vi "DO State Machine.vi"(0 "DO in":bool, 5 "Set":bool, 7 "Time uSec":u32) -> (4 "DO out":bool)   [LabVIEW 2019]
uses:
  <vilib>/rvi/Emulation/niFpgaGetClockAttributes.vi
  <vilib>/rvi/Emulation/niFpgaSctlEmulationGetInTimedLoop.vi
  <vilib>/rvi/Emulation/niFpgaEmulationReportErrorSimple.vi
  <vilib>/rvi/Emulation/niFpgaCriticalErrorInLSC.vi
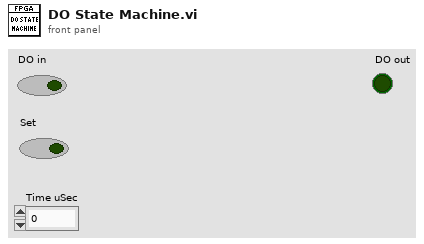
[diagram p1: front panel]
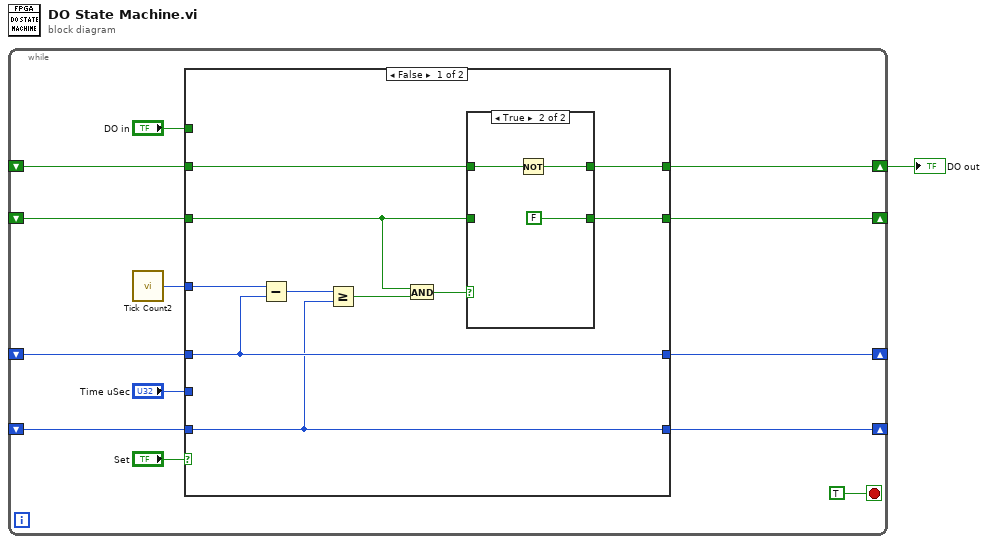
[diagram p0: block diagram]
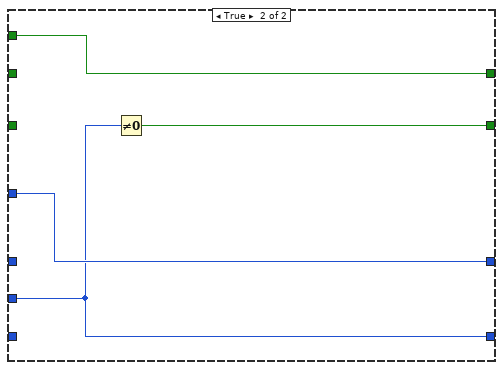
[diagram p3: hidden frame]
diagram:
  n1 = while {
    shift-right: [w9] -> _
    shift-left: _ -> [w8]
    shift-right: [w7] -> _
    shift-left: _ -> [w4]
    shift-right: [w6] -> w1
    shift-left: _ -> [w5]
    shift-right: [w3] -> _
    shift-left: _ -> [w2]
    stop <- TRUE stop-if-true
    n2 = call "Tick Count2"() -> ("Tick Count(uSec)"=w11:u32)
    n3 = case shown="False" "Set" {
      tunnel: "DO in" -> [_ w33]
      tunnel: [w19 w33] -> w6
      tunnel: w5 -> [w20 _]
      tunnel: "Time uSec" -> [_ w31]
      tunnel: w11 -> [w24 w32]
      tunnel: [w22 w32] -> w9
      tunnel: w8 -> [w22 _]
      tunnel: [w21 w31] -> w7
      tunnel: w4 -> [w21 _]
      tunnel: [w18 w30] -> w3
      tunnel: w2 -> [w15 _]
      frame False {
        n4 = Subtract(x=w24, y=w22) -> (x-y=w23:u32)
        n5 = Greater Or Equal?(x=w23, y=w21) -> (x >= y?=w16:bool)
        n6 = And(x=w15, y=w16) -> (x .and. y?=w17:bool)
        n7 = case shown="True" w17 {
          tunnel: w20 -> [w26 w29]
          tunnel: [w26 w28] -> w19
          tunnel: [w25 FALSE] -> w18
          tunnel: w15 -> [w25 _]
          frame False {
          }
          frame True {
            n8 = Not(x=w29) -> (.not. x?=w28:bool)
          }
        }
      }
      frame True {
        n9 = Not Equal To 0?(x=w31) -> (x != 0?=w30:bool)
      }
    }
  }
  "DO out" <- w1
